vi "Buffer Profiles.vi"(0 "Buffer for Batch Profile\n(before buffering)":u32[](array[numeric]), 5 "Bufferd Profile Cnt\n(before buffering)":u32, 7 "Profile Data":u32[](array[numeric]), 9 "Profile Info":T2, 11 "Profile Rsp":T1) -> (4 ">Buffer for Batch Profile\n (after buffering) >":u32[](array[numeric]), 6 ">Bufferd Profile Cnt\n (after buffering)>":u32)   [LabVIEW 2014]
uses:
  Public/Clusters/Profile Info.ctl
  Public/Clusters/Read Batch Profile Rsp.ctl
  Keyence LJ-V7000.lvlib
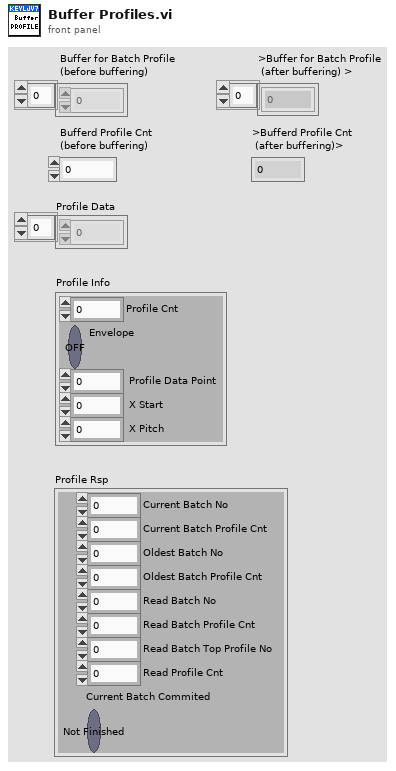
[diagram p1: front panel]
types:
  T1 = typedef "Keyence LJ-V7000.lvlib/Read Batch Profile Rsp.ctl" = cluster{"Current Batch No":u32, "Current Batch Profile Cnt":u32, "Oldest Batch No":u32, "Oldest Batch Profile Cnt":u32, "Read Batch No":u32, "Read Batch Profile Cnt":u32, "Read Batch Top Profile No":u32, "Read Profile Cnt":u8, "Current Batch Commited":bool}
  T2 = typedef "Keyence LJ-V7000.lvlib/Profile Info.ctl" = cluster{"Profile Cnt":u8, "Envelope":bool, " Profile Data Point":u16, " X Start":i32, " X Pitch":i32}
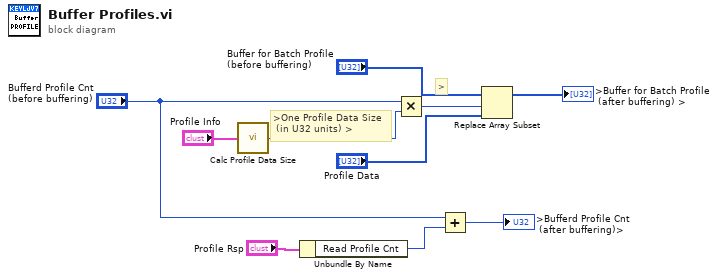
[diagram p0: block diagram]
diagram:
  # ">"
  # ">One Profile Data Size\n (in U32 units) >"
  n1 = call "Calc Profile Data Size.vi"("Profile Info"="Profile Info") -> ("Profile Data Size in U32"=w4:u32)  [unwired: 4 in]
  n2 = Unbundle By Name("Profile Rsp") -> ("Read Profile Cnt"=w1:u8)
  n3 = Multiply(x="Bufferd Profile Cnt\n(before buffering)", y=w4) -> (x*y=w3:u32)
  n4 = Add(x="Bufferd Profile Cnt\n(before buffering)", y=w1) -> (x+y=→">Bufferd Profile Cnt\n (after buffering)>":u32)
  n5 = Replace Array Subset(array="Buffer for Batch Profile\n(before buffering)", new element="Profile Data", index=w3) -> (→">Buffer for Batch Profile\n (after buffering) >":u32[])
